vi "Is_InSpec.vi"(1 "HRI_Lum_Max":dbl, 2 "HRI_Lum_Min":dbl, 3 "InputNumeric":dbl) -> (0 "Boolean":bool)   [LabVIEW 2014]
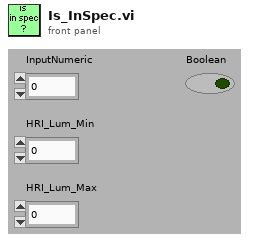
[diagram p1: front panel]
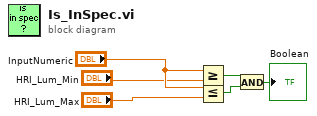
[diagram p0: block diagram]
diagram:
  n1 = Greater Or Equal?(x="InputNumeric", y="HRI_Lum_Min") -> (x >= y?=w4:bool)
  n2 = Less Or Equal?(x="InputNumeric", y="HRI_Lum_Max") -> (x <= y?=w5:bool)
  n3 = And(x=w4, y=w5) -> (x .and. y?=→"Boolean":bool)
